vi "运维调试_总氮.vi"() -> ()   [LabVIEW 2016, in "斯坦道总氮.lvlib"]
uses:
  <vilib>/Utility/miscctls.llb/LVPointTypeDef.ctl
  <vilib>/Utility/config.llb/NI_LVConfig.lvlib
  <vilib>/ptbypt/NI_PtbyPt.lvlib
panel:
  in  "定时设置":cluster{"启动":bool, "控制命令":T1}(xcontrol)
  out "单位:":T2(ring)
  out "模块版本号":string
  in  "校准按钮":T3
  out "运行状态":T4 {"数据时间:" format="%<%y/%m/%d %H:%M:%S>T"; "仪器时间:" format="%<%y/%m/%d %H:%M:%S>T"}
  out "一级权限":bool
  out "二级权限":bool
  out "输入密码":u32
  out "布尔":bool
  in  "流程固件":bool
  in  "仪器参数设置":bool
  in  "量程参数读取":T5
  in  "模块启用":bool
  in  "串口设置":bool
  in  "公式一键写入":bool
  in  "流程路径":path=path "C:/Users/STD/Documents/斯坦道流程文件/流程.xml"
  in  "曲线模型":cluster{"X^2":dbl, "X":dbl, "B":dbl, "r^2":dbl}(xcontrol)
  out "字符串":string
  in  "质控参数设置":bool
  in  "自动测试量程配置":T6
  out "温度2":sgl
  out "温度1":sgl
  out "ADC":sgl
  out "固件版本号":string
  in  "数组":string[](array[string])
  in  "量程切换阈值写入":bool
  in  "量程切换阈值读取":bool
  in  "参数下拉列表":enum16{"总磷", "总氮"}(ring)=enum."总氮"
  in  "量程下拉列表":enum16{"低量程", "高量程"}(ring)
  in  "测量模式下拉列表":enum16{"水样测量", "零点核查", "跨度核查", "标样核查", "加标回收"}(ring)
  in  "公式":cluster{"X^2":dbl, "X":dbl, "b":dbl}
  in  "写公式":bool
  in  "读公式":bool
  in  "返回":bool
  in  "设置":bool
  out "集成报警信息":string
  in  "停止":bool
  in  "手动启动":bool
  in  "单步测试":bool
  out "F3":sgl format="%#.6f"
  out "F2":sgl format="%#.6f"
  out "F1":sgl format="%#.6f"
  out "F0":sgl format="%#.6f"
  out "多列列表框":i32(listbox)
  # "参数设置"
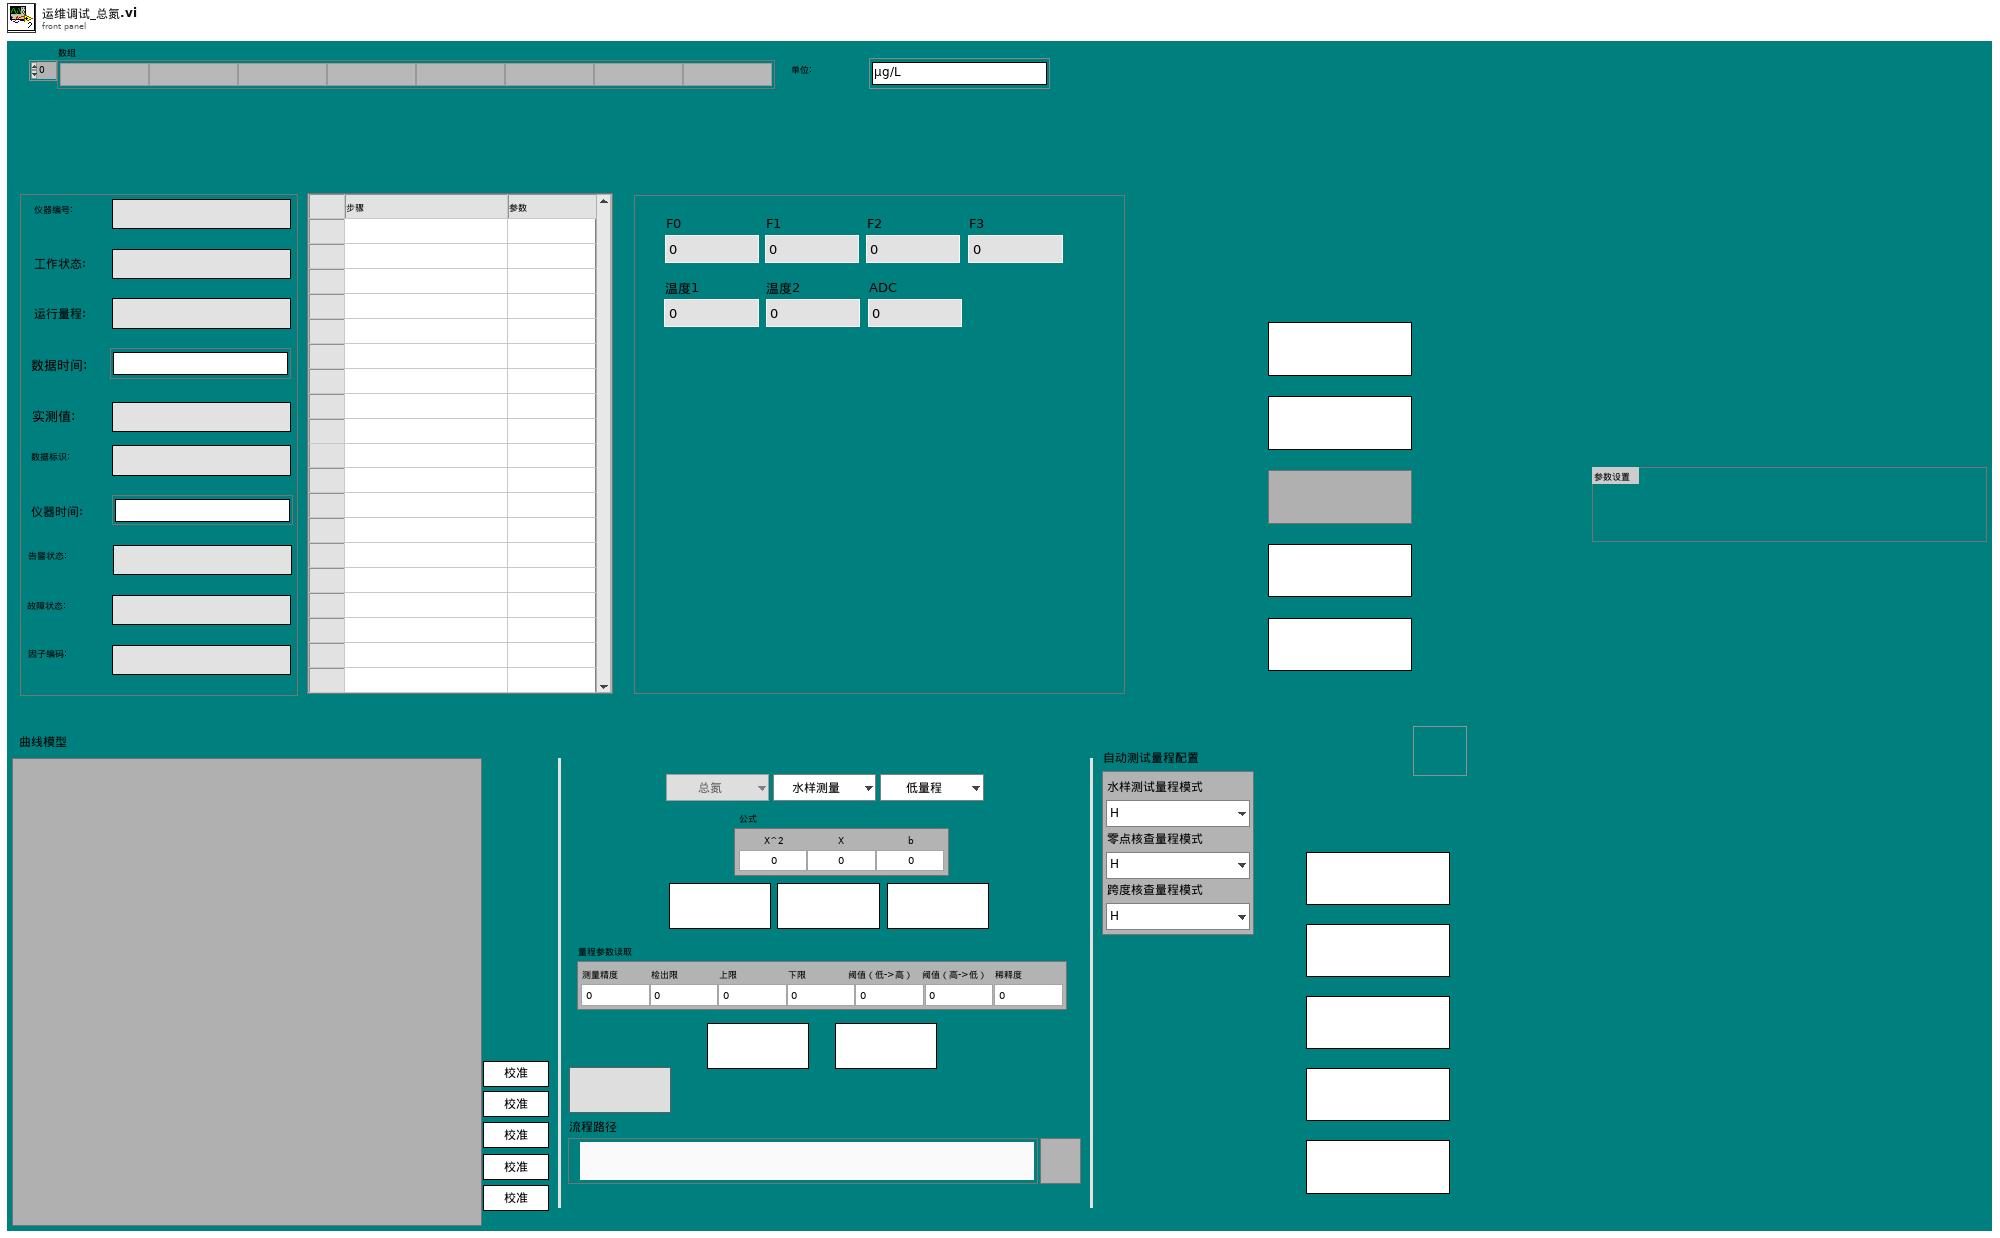
[diagram p1: front panel]
types:
  T1 = typedef "定时设置.xctl/国标控制命令.ctl" = enum16{"启动测量", "标样核查", "零点核查", "跨度核查", "空白测试", "平行样测试", "加标回收", "空白校准", "标样校准", "初始化（清洗）", "停止测试", "仪器重启", "校时", "模式设置", "测量间隔设置"}
  T2 = enum16{"μg/L", "mg/L", "ppm", "mg/m3", "cm", "ppb", "μg/m3", "%", "nmol/mol", "μmol/mol", "MPN/L", "MPN/100ml", "ng/m3", "NTU", "无量纲", "mS/cm", "μS/cm", "℃", "mV", "cells/mL"}
  T3 = cluster{"校准1":bool, "校准2":bool, "校准3":bool, "校准4":bool, "校准5":bool}
  T4 = cluster{"仪器编号:":string, "工作状态:":string, "运行量程: ":string, "数据时间:":timestamp, "实测值:":string, "数据标识: ":string, "仪器时间:":timestamp, "告警状态: ":string, "故障状态:  ":string, "因子编码:":string}
  T5 = cluster{"测量精度":dbl, "检出限":dbl, "上限":dbl, "下限":dbl, "阈值（低->高）":dbl, "阈值（高->低）":dbl, "稀释度":dbl}
  T6 = cluster{"水样测试量程模式":enum16{"H", "L", "AUTO"}, "空白核查量程模式":enum16{"H", "L", "AUTO"}, "跨度核查量程模式":enum16{"H", "L", "AUTO"}}
  T7 = typedef "LVPointTypeDef.ctl" = cluster{"Horizontal":i16, "Vertical":i16}
  T8 = cluster{"系统时间":timestamp, "工作状态":enum16{"空闲", "水样测试", "标样核查", "零点核查", "跨度核查", "空白测试", "平行样测试", "加标回收", "空白校准", "标样校准", "初始化（清洗）"}, "测量模式":enum16{"待机", "连续模式", "周期模式", "定点模式", "受控模式", "手动模式"}, "告警代码":u16, "故障代码":u16, "日志代码":u16, "软件版本":u16, "F0":sgl, "F1":sgl, "F2":sgl, "F3":sgl, "T":sgl, "H":sgl, "id":u16, "flowid":u16, "量程":u16, "总磷控温温度1":sgl, "营养盐控温温度2":sgl, "ADC":sgl}
  T9 = cluster{"因子编码":u32, "单位":u16, "标样参考值":sgl, "水样数据时间":timestamp, "水样实测值":sgl, "水样数据标识":string, "标样数据时间":timestamp, "标样实测值":sgl, "标样数据标识":string, "空白数据时间":timestamp, "空白实测值":sgl, "空白数据标识":string, "零点核查数据时间":timestamp, "零点核查实测值":sgl, "零点核查数据标识":string, "跨度核查数据时间":timestamp, "跨度核查实测值":sgl, "跨度核查数据标识":string, "加标回收数据时间":timestamp, "加标回收实测值":sgl, "加标回收数据标识":string, "平行样数据时间":timestamp, "平行样实测值":sgl, "平行样数据标识":string, "F0":sgl, "F1":sgl, "F2":sgl, "F3":sgl, "F4":sgl, "F5":sgl, "F6":sgl, "F7":sgl, "温度":sgl, "湿度":sgl, "X值":sgl, "fidrange":u16}
  T10 = enum16{"空闲", "水样测试", "标样核查", "零点核查", "跨度核查", "空白测试", "平行样测试", "加标回收", "空白校准", "标样校准", "初始化（清洗）"}
  T11 = enum8{"Enabled", "Disabled", "Disabled and Grayed Out"}
  T12 = cluster{"参数下拉列表":enum16{"总磷", "总氮"}, "测量模式下拉列表":enum16{"水样测量", "零点核查", "跨度核查", "标样核查", "加标回收"}, "量程下拉列表":enum16{"低量程", "高量程"}}
  T13 = cluster{"Major":u16, "Minor":u16, "Fix":u16, "Build":u16}
  T14 = typedef "NI_LVConfig.lvlib/Config Data RefNum.ctl" = refnum<k1>
  T15 = cluster{"启动模式":enum16{"跨度核查", "水样测量", "空白核查", "标样核查", "加标回收"}, "启动参数":u16, "量程":enum16{"低量程", "高量程"}}
  T16 = cluster{"时间标识":timestamp, "设备":string, "日志信息":string, "流程参数":string}
  T17 = typedef "LVRowAndColumnUnsignedTypeDef.ctl" = cluster{"Row":u32, "Column":u32}
  T18 = cluster{"站号":u16, "量程切换":enum32{"H", "L", "AUTO"}, "控制命令":enum16{"启动测量", "标样核查", "零点核查", "跨度核查", "空白测试", "平行样测试", "加标回收", "空白校准", "标样校准", "初始化（清洗）", "停止测试", "仪器重启", "校时", "模式设置", "测量间隔设置"}, "模式设置":enum16{"待机", "连续模式", "周期模式", "定点模式", "受控模式", "手动模式"}, "测量间隔":u16}
  T19 = cluster{"跨度值":dbl, "零点标准液浓度":dbl, "跨度标准液浓度":dbl, "标准液标准浓度":dbl}
  T20 = cluster{"确定":bool, "跨度值":dbl, "零点标准液浓度":dbl, "跨度标准液浓度":dbl, "标准液标准浓度":dbl}
  T21 = cluster{"测量量程":dbl, "测量精度":dbl, "测量间隔":dbl, "消解温度":dbl, "消解时长":dbl, "空白校准时间":timestamp, "曲线截距":dbl, "曲线斜率":dbl, "测量检出限":dbl, "测量信号值":dbl, "线性相关系数":dbl, "二次多项式系数":dbl, "标样校准时间":timestamp, "稀释倍数":dbl, "三项式系数":dbl, "空白标定系数":dbl, "量程系数":dbl, "F0/ORPA":dbl, "F1/ORPB":dbl, "F2/ORPK":dbl, "F3":dbl, "F4":dbl, "F5":dbl, "F6":dbl, "F7":dbl, "X0/滴定数":dbl, "量程":dbl}
  T22 = cluster{"确定":bool, "测量量程":dbl, "测量精度":dbl, "测量间隔":dbl, "消解温度":dbl, "消解时长":dbl, "空白校准时间":timestamp, "曲线截距":dbl, "曲线斜率":dbl, "测量检出限":dbl, "测量信号值":dbl, "线性相关系数":dbl, "二次多项式系数":dbl, "标样校准时间":timestamp, "稀释倍数":dbl, "三项式系数":dbl, "空白标定系数":dbl, "量程系数":dbl, "F0/ORPA":dbl, "F1/ORPB":dbl, "F2/ORPK":dbl, "F3":dbl, "F4":dbl, "F5":dbl, "F6":dbl, "F7":dbl, "X0/滴定数":dbl, "量程":dbl}
  T23 = cluster{"标液浓度1":dbl, "标液浓度2":dbl, "标液浓度3":dbl, "标液浓度4":dbl, "标液浓度5":dbl}
  T24 = cluster{"测量精度":u16, "检出限":dbl, "上限":dbl, "下限":dbl, "阈值（低->高）":dbl, "阈值（高->低）":dbl, "稀释度":dbl}
  T25 = enum32{"Bad", "Idle", "Run top level", "Running"}
  T26 = typedef "定时设置.xctl/周期模式设置.ctl" = enum16{"不启用", "定点模式", "间隔模式"}
  T27 = typedef "定时设置.xctl/定点周期设置.ctl" = cluster{"启动命令":T28, "启动命令 2":T28, "启动命令 3":T28, "启动命令 4":T28, "启动命令 5":T28, "启动命令 6":T28, "启动命令 7":T28, "启动命令 8":T28, "启动命令 9":T28, "启动命令 10":T28, "启动命令 11":T28, "启动命令 12":T28, "启动命令 13":T28, "启动命令 14":T28, "启动命令 15":T28, "启动命令 16":T28, "启动命令 17":T28, "启动命令 18":T28, "启动命令 19":T28, "启动命令 20":T28, "启动命令 21":T28, "启动命令 22":T28, "启动命令 23":T28, "启动命令 24":T28}
  T28 = typedef "定时设置.xctl/启动命令选择.ctl" = u16
  T29 = typedef "定时设置.xctl/间隔启动设置.ctl" = cluster{"启动命令":T28, "启动间隔":dbl, "启动次数":i32}
  T30 = cluster{"时间标识":timestamp, "设备":string, "日志信息":string, "备注":string}
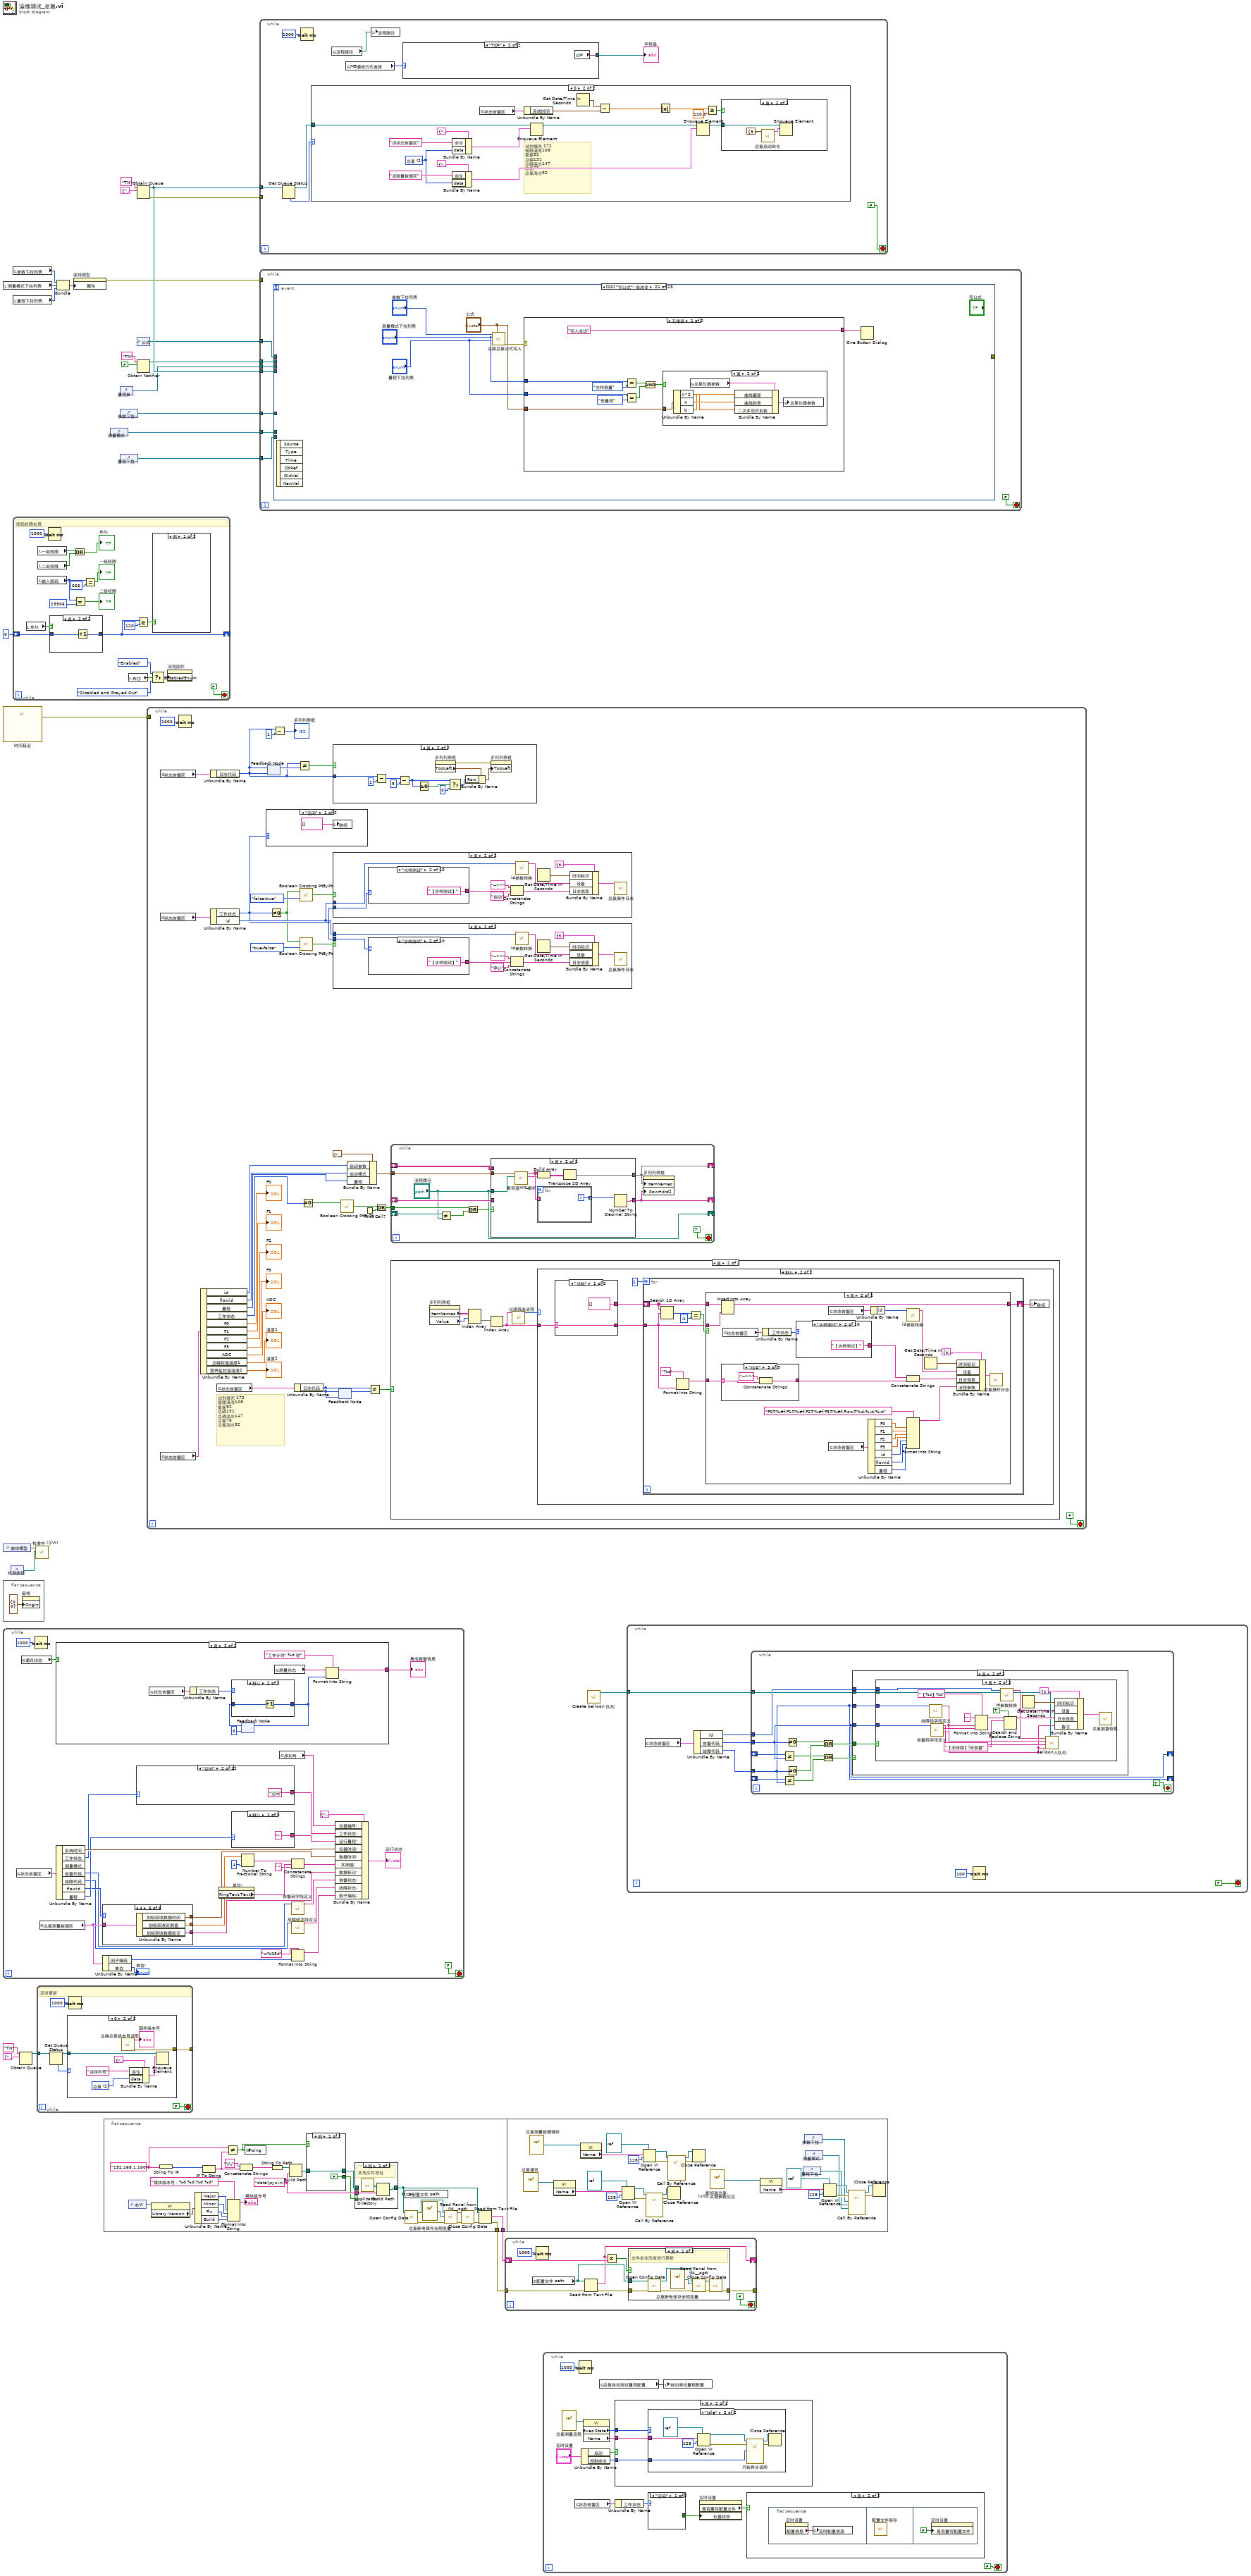
[diagram p0: block diagram]
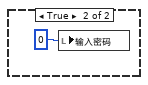
[diagram p5: hidden frame]
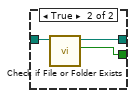
[diagram p7: hidden frame]
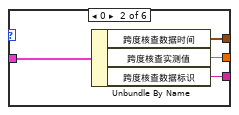
[diagram p11: hidden frame]
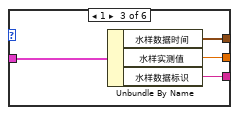
[diagram p12: hidden frame]
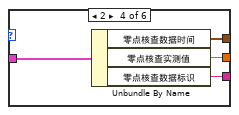
[diagram p13: hidden frame]
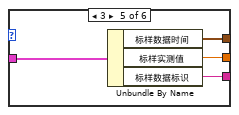
[diagram p14: hidden frame]
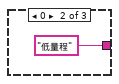
[diagram p15: hidden frame]
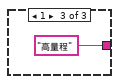
[diagram p16: hidden frame]
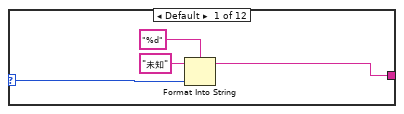
[diagram p17: hidden frame]
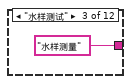
[diagram p18: hidden frame]
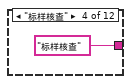
[diagram p19: hidden frame]
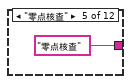
[diagram p20: hidden frame]
diagram:
  n1 = local read "测量模式下拉列表"() -> (w9:enum16{"水样测量", "零点核查", "跨度核查", "标样核查", "加标回收"})
  n2 = call "时间延迟"() -> ("error out"=w19:errorcluster)  [unwired: 11 in]
  n3 = control-ref of="曲线模型"() -> (w4:refnum<vi>)
  n4 = flat-sequence {
    frame #0 {
      n5 = property on="窗格" class="Pane"("Origin"=T7 {"Horizontal"=0, "Vertical"=0} ("原点")) -> ()  [unwired: 2 in, 2 out]
    }
  }
  n6 = while {
    stop <- FALSE stop-if-true
    n7 = global read "VAR总氮全局变量.vi" "状态告警区"() -> (w49:T8)
    n8 = global read "VAR总氮全局变量.vi" "通讯状态"() -> (w57:bool)
    n9 = Wait (ms)(milliseconds to wait=u32 1000 ("等待时间（毫秒）")) -> ()  [unwired: 1 out]
    n10 = global read "VAR总氮全局变量.vi" "总氮测量数据区"() -> (w46:T9)
    n11 = case shown="真" w57 {
      tunnel: ["通讯异常" ("集成报警信息") w100] -> w56
      frame False {
      }
      frame True {
        n12 = global read "VAR总氮全局变量.vi" "状态告警区"() -> (w106:T8)
        n13 = Unbundle By Name(w106) -> ("工作状态"=w105:T10)
        n14 = feedback #1(0) -> (w103:i32)
        n15 = case shown="默认" w105 {
          tunnel: w103 -> [_ w108]
          tunnel: [_ w107] -> w101
          frame "空闲" {
          }
          frame Default {
            n16 = Increment(x=w108) -> (x+1=w107:i32)
          }
        }
        n17 = feedback-in #1(w101) -> ()
        n18 = global read "VAR总氮全局变量.vi" "测量状态"() -> (w99:string)
        n19 = Format Into String(format string="工作计时: %d 秒" ("格式字符串"), initial string=w99, w101) -> (resulting string=w100:string)  [unwired: 1 in, 1 out]
      }
    }
    "集成报警信息" <- w56
    n20 = Unbundle By Name(w49) -> ("系统时间"=w55:timestamp, "工作状态"=w47:T10, "告警代码"=w32:u16, "故障代码"=w30:u16, "flowid"=w45:u16, "量程"=w53:u16)  [unwired: 1 out]
    n21 = case shown="4" w45 {
      tunnel: [_ w63 w67 w71 w75 w79] -> w41
      tunnel: [_ w61 w66 w70 w74 w78] -> w37
      tunnel: [_ w60 w65 w69 w73 w77] -> w34
      tunnel: w46 -> [_ w62 w64 w68 w72 w76]
      frame Default {
      }
      frame 0 {
        n22 = Unbundle By Name(w62) -> ("跨度核查数据时间"=w63:timestamp, "跨度核查实测值"=w61:sgl, "跨度核查数据标识"=w60:string)
      }
      frame 1 {
        n23 = Unbundle By Name(w64) -> ("水样数据时间"=w67:timestamp, "水样实测值"=w66:sgl, "水样数据标识"=w65:string)
      }
      frame 2 {
        n24 = Unbundle By Name(w68) -> ("零点核查数据时间"=w71:timestamp, "零点核查实测值"=w70:sgl, "零点核查数据标识"=w69:string)
      }
      frame 3 {
        n25 = Unbundle By Name(w72) -> ("标样数据时间"=w75:timestamp, "标样实测值"=w74:sgl, "标样数据标识"=w73:string)
      }
      frame 4 {
        n26 = Unbundle By Name(w76) -> ("加标回收数据时间"=w79:timestamp, "加标回收实测值"=w78:sgl, "加标回收数据标识"=w77:string)
      }
    }
    n27 = Unbundle By Name(w46) -> ("因子编码"=w50:u32, "单位"=→"单位:":u16)
    n28 = case shown="\"空闲\"" w47 {
      selector: w47 -> [w83 _ _ _ _ _ _ _ _ _ _ _]
      tunnel: [w84 "空闲" ("工作状态") "水样测量" ("工作状态") "标样核查" ("工作状态") "零点核查" ("工作状态") "跨度核查" ("工作状态") "空白测试" ("工作状态") "平行样测试" ("工作状态") "加标回收" ("工作状态") "空白校准" ("工作状态") "标样校准" ("工作状态") "初始化" ("工作状态")] -> w54
      frame Default {
        n29 = Format Into String(format string="%d" ("格式字符串"), initial string="未知" ("工作状态"), w83) -> (resulting string=w84:string)  [unwired: 1 in, 1 out]
      }
      frame "空闲" {
      }
      frame "水样测试" {
      }
      frame "标样核查" {
      }
      frame "零点核查" {
      }
      frame "跨度核查" {
      }
      frame "空白测试" {
      }
      frame "平行样测试" {
      }
      frame "加标回收" {
      }
      frame "空白校准" {
      }
      frame "标样校准" {
      }
      frame "初始化（清洗）" {
      }
    }
    n30 = property on="单位:" class="Enum (严格)"() -> ("RingText.Text"=w38:string)  [unwired: 2 in, 2 out]
    n31 = case shown="默认" w53 {
      tunnel: ["" ("字符串") "低量程" ("字符串") "高量程" ("字符串")] -> w52
      frame Default {
      }
      frame 0 {
      }
      frame 1 {
      }
    }
    n32 = Number To Fractional String(number=w37, precision (6)=i16 4 ("精度(6)")) -> (F-format string=w36:string)  [unwired: 2 in]
    n33 = global read "VAR总氮全局变量.vi" "序列号"() -> (w48:string)
    n34 = Concatenate Strings(w36, " " ("字符串"), w38) -> (w35:string)
    n35 = call "告警码字段定义.vi"("告警代码"=w32) -> ("字符串"=w31:string)  [unwired: 8 in, 2 out]
    n36 = call "故障码字段定义.vi"("故障代码"=w30) -> ("字符串"=w29:string)  [unwired: 10 in]
    n37 = Format Into String(format string="w%05d" ("格式字符串"), w50) -> (resulting string=w33:string)  [unwired: 2 in, 1 out]
    n38 = Bundle By Name(cluster=T4 {"仪器编号:"="", "工作状态:"="", "运行量程: "="", "数据时间:"=timestamp(0 s since 1904-01-01), "实测值:"="", "数据标识: "="", "仪器时间:"=timestamp(0 s since 1904-01-01), "告警状态: "="", "故障状态:  "="", "因子编码:"=""} ("运行状态"), "仪器编号:"=w48, "工作状态:"=w54, "运行量程:"=w52, "仪器时间:"=w55, "数据时间:"=w41, "实测值:"=w35, "数据标识:"=w34, "告警状态:"=w31, "故障状态:"=w29, "因子编码:"=w33) -> (→"运行状态":T4)
  }
  n39 = control-ref of="校准按钮"() -> (w3:refnum<vi>)
  n40 = local read "参数下拉列表"() -> (w10:enum16{"总磷", "总氮"})
  n41 = local read "量程下拉列表"() -> (w8:enum16{"低量程", "高量程"})
  n42 = while {
    shift-right: [w115] -> _
    shift-left: u32 0 ("等待时间（毫秒）") -> [w116]
    stop <- FALSE stop-if-true
    # "密码权限处理"
    n43 = local read "布尔"() -> (w117:bool)
    n44 = local read "一级权限"() -> (w119:bool)
    n45 = local read "二级权限"() -> (w120:bool)
    n46 = local read "输入密码"() -> (w123:u32)
    n47 = Wait (ms)(milliseconds to wait=u32 1000 ("等待时间（毫秒）")) -> ()  [unwired: 1 out]
    n48 = case shown="真" w117 {
      tunnel: w116 -> [_ w130]
      tunnel: [_ w129] -> w115
      frame False {
      }
      frame True {
        n49 = Increment(x=w130) -> (x+1=w129:u32)
      }
    }
    n50 = Or(x=w119, y=w120) -> (x .or. y?=→"布尔":bool)
    n51 = Equal?(x=w123, y=u32 23506) -> (x = y?=→"二级权限":bool)
    n52 = Equal?(x=w123, y=u32 666) -> (x = y?=→"一级权限":bool)
    n53 = local read "布尔"() -> (w112:bool)
    n54 = Greater Or Equal?(x=w115, y=u32 120) -> (x >= y?=w113:bool)
    n55 = Select(t=T11."Enabled" ("禁用"), s=w112, f=T11."Disabled and Grayed Out") -> (s? t:f=w110:T11)
    n56 = case shown="假" w113 {
      frame False {
      }
      frame True {
        n57 = local write "输入密码"(u32 0 ("输入密码")) -> ()
      }
    }
    n58 = property on="流程固件" class="Bool"("DisabledEnum"=w110) -> ()  [unwired: 2 in, 2 out]
  }
  n59 = Obtain Queue(name (unnamed)="TN" ("名称（未命名）"), element data type=cluster{"命令":string, "data":variant} {"命令"="", "data"=variant}) -> (queue out=w16:refnum<queue>)  [unwired: 3 in, 2 out]
  n60 = call "校准中 (子VI).vi"("曲线模型"=w4, "校准按钮"=w3) -> ()  [unwired: 9 in]
  n61 = while {
    tunnel: w16 -> [w135]
    tunnel: [w133] -> _
    stop <- FALSE stop-if-true
    # "定时更新"
    n62 = Get Queue Status(queue=w135) -> (queue out=w132:refnum<queue>, # elements in queue=w131:i32)  [unwired: 2 in, 6 out]
    n63 = case shown="0" w131 {
      tunnel: [_ w138] -> w133
      tunnel: w132 -> [_ w137]
      frame Default {
      }
      frame 0 {
        w141 = u16 2 items=["总磷"=1, "总氮"=2, "氨氮"=3] ("站号")
        n64 = call "总磷总氮版本号读取.vi"() -> ("error out"=w138:errorcluster, "固件版本号"=→"固件版本号":string)  [unwired: 10 in]
        n65 = Bundle By Name(cluster=cluster{"命令":string, "data":variant} {"命令"="", "data"=variant} ("元素"), "命令"="读序列号", "data"=w141) -> (w140:cluster{"命令":string, "data":variant})
        n66 = Enqueue Element(queue=w137, element=w140) -> ()  [unwired: 2 in, 3 out]
      }
    }
    n67 = Wait (ms)(milliseconds to wait=u32 1000 ("等待时间（毫秒）")) -> ()  [unwired: 1 out]
  }
  n68 = Bundle("参数下拉列表"=w10, "测量模式下拉列表"=w9, "量程下拉列表"=w8) -> (w7:T12)  [unwired: 1 in]
  n69 = property on="曲线模型" class="曲线模型 (严格)"("属性"=w7) -> (error out=w15:errorcluster)  [unwired: 2 in, 1 out]
  n70 = flat-sequence {
    tunnel: [w153] -> w1
    tunnel: [w152] -> w5
    frame #0 {
      w166 = "data\\sys.ini" ("名称或相对路径")
      w158 = "192.168.1.100" ("名称")
      n71 = control-ref of="本VI"() -> (w151:refnum<vi>)
      n72 = property class="VI"(reference=w151) -> ("Library.Version"=w150:T13)  [unwired: 1 in, 2 out]
      n73 = String To IP(1:w158) -> (0:w165:u32)
      n74 = Unbundle By Name(w150) -> ("Major"=w148:u16, "Minor"=w147:u16, "Fix"=w146:u16, "Build"=w145:u16)
      n75 = IP To String(2:w165) -> (0:w162:string)  [unwired: 1 in]
      n76 = Not Equal?(x=w158, y=w162) -> (x != y?=w156:bool)
      n77 = Format Into String(format string="模块版本号：%d.%d.%d.%d" ("格式字符串"), w148, w147, w146, w145) -> (resulting string=→"模块版本号":string)  [unwired: 2 in, 1 out]
      n78 = Concatenate Strings("\\\\" ("字符串"), w162) -> (w163:string)
      n79 = global write "VAR总氮全局变量.vi" "ping"(w156) -> ()
      n80 = String To Path(string=w163) -> (path=w157:path)
      n81 = Build Path(base path=w157, name or relative path=w166) -> (appended path=w161:path)
      n82 = case shown="假" w156 {
        tunnel: w161 -> [w172 w176]
        tunnel: [w172 w175] -> w160
        tunnel: [FALSE w174] -> w159
        frame False {
        }
        frame True {
          n83 = call <vilib>:"Check if File or Folder Exists.vi"("path"=w176) -> ("file or folder exists?"=w174:bool, "dup path"=w175:path)  [unwired: 8 in, 1 out]
        }
      }
      n84 = case shown="假" w159 {
        tunnel: w160 -> [_ w180]
        tunnel: [w178 w180] -> w155
        tunnel: w166 -> [w177 _]
        frame False {
          # "本地文件地址"
          n85 = call <vilib>:"Application Directory.vi"() -> ("Application Directory"=w179:path)
          n86 = Build Path(base path=w179, name or relative path=w177) -> (appended path=w178:path)
        }
        frame True {
          # "网络共享地址"
        }
      }
      n87 = global write "VAR总氮全局变量.vi" "配置文件 path"(w155) -> ()
      n88 = call <vilib>:"Open Config Data.vi"("configuration file path"=w155) -> ("error out"=w168:errorcluster, "refnum"=w171:T14)  [unwired: 8 in, 1 out]
      n89 = vi-ref "总氮断电保存全局变量.vi"() -> (w170:refnum<vi>)
      n90 = call <userlib>:"Read Panel from INI__ogtk.vi"("error in (no error)"=w168, "VI ref"=w170, "refnum"=w171) -> ("error out"=w167:errorcluster, "refnum out"=w169:T14)  [unwired: 7 in]
      n91 = call <vilib>:"Close Config Data.vi"("error in (no error)"=w167, "refnum"=w169) -> ("error out"=w154:errorcluster)  [unwired: 8 in, 1 out]
      n92 = Read from Text File(file (use dialog)=w155, error in=w154) -> (text=w152:string, error out=w153:errorcluster)  [unwired: 2 in, 2 out]
    }
    frame #1 {
      n93 = vi-ref "总氮通讯.vi"() -> (w207:refnum<vi>)
      n94 = vi-ref "总氮测量数据储存.vi"() -> (w199:refnum<vi>)
      n95 = property class="VI"(reference=w207) -> ("Name"=w206:string)  [unwired: 1 in, 2 out]
      n96 = property class="VI"(reference=w199) -> ("Name"=w192:string)  [unwired: 1 in, 2 out]
      n97 = Open VI Reference(type specifier VI Refnum (for type only)=refnum<vi> refnum, vi path=w206, options=128 ("选项")) -> (vi reference=w204:refnum<vi>, error out=w202:errorcluster)  [unwired: 3 in]
      n98 = Open VI Reference(type specifier VI Refnum (for type only)=refnum<vi> refnum, vi path=w192, options=128 ("选项")) -> (vi reference=w194:refnum<vi>, error out=w196:errorcluster)  [unwired: 3 in]
      n99 = call-by-ref "?"(reference=w204, error in=w202) -> (reference out=w200:refnum<vi>, error out=w201:errorcluster)  [unwired: 12 in]
      n100 = call-by-ref "?"(reference=w194, error in=w196) -> (reference out=w198:refnum<vi>, error out=w197:errorcluster)  [unwired: 12 in]
      n101 = Close Reference(reference=w200, error in (no error)=w201) -> ()  [unwired: 1 out]
      n102 = Close Reference(reference=w198, error in (no error)=w197) -> ()  [unwired: 1 out]
      n103 = vi-ref "斯坦道总氮.lvlib:关键参数交互.vi"() -> (w184:refnum<vi>)
      n104 = property class="VI"(reference=w184) -> ("Name"=w191:string)  [unwired: 1 in, 2 out]
      n105 = control-ref of="量程下拉列表"() -> (w181:refnum<vi>)
      n106 = control-ref of="参数下拉列表"() -> (w183:refnum<vi>)
      n107 = control-ref of="测量模式下拉列表"() -> (w182:refnum<vi>)
      n108 = Open VI Reference(type specifier VI Refnum (for type only)=refnum<vi> refnum, vi path=w191, options=128 ("选项")) -> (vi reference=w189:refnum<vi>, error out=w187:errorcluster)  [unwired: 3 in]
      n109 = call-by-ref "?"(reference=w189, error in=w187, "量程下拉列表"=w181, "测量模式下拉列表"=w182, "测量参数"=w183) -> (reference out=w185:refnum<vi>, error out=w186:errorcluster)  [unwired: 9 in]
      n110 = Close Reference(reference=w185, error in (no error)=w186) -> ()  [unwired: 1 out]
    }
  }
  n111 = control-ref of="测量模式下拉列表"() -> (w21:refnum<vi>)
  n112 = control-ref of="量程参数读取"() -> (w11:refnum<vi>)
  n113 = control-ref of="参数下拉列表"() -> (w22:refnum<vi>)
  n114 = control-ref of="量程下拉列表"() -> (w23:refnum<vi>)
  n115 = Obtain Queue(name (unnamed)="TN" ("名称（未命名）"), element data type=cluster{"命令":string, "data":variant} {"命令"="", "data"=variant}) -> (queue out=w24:refnum<queue>, error out=w25:errorcluster)  [unwired: 3 in, 1 out]
  n116 = control-ref of="公式"() -> (w20:refnum<vi>)
  n117 = Obtain Notifier(name (unnamed)="TN" ("名称（未命名）"), notification data type=FALSE) -> (notifier out=w12:refnum<notifier>)  [unwired: 2 in, 2 out]
  n118 = while {
    tunnel: w19 -> [_]
    stop <- FALSE stop-if-true
    # "试剂填充 172 \n管路清洗108\n氨氮92\n总磷131\n总磷海水147\n总氮76\n总氮海水92"
    n119 = global read "VAR总氮全局变量.vi" "状态告警区"() -> (w230:T8)
    n120 = global read "VAR总氮全局变量.vi" "状态告警区"() -> (w228:T8)
    n121 = global read "VAR总氮全局变量.vi" "状态告警区"() -> (w238:T8)
    n122 = Wait (ms)(milliseconds to wait=u32 1000 ("等待时间（毫秒）")) -> ()  [unwired: 1 out]
    n123 = Unbundle By Name(w238) -> ("id"=w235:u16, "flowid"=w237:u16, "量程"=w236:u16, "工作状态"=w216:T10, "F0"=→"F0":sgl, "F1"=→"F1":sgl, "F2"=→"F2":sgl, "F3"=→"F3":sgl, "ADC"=→"ADC":sgl, "总磷控温温度1"=→"温度1":sgl, "营养盐控温温度2"=→"温度2":sgl)
    n124 = Unbundle By Name(w230) -> ("日志代码"=w222:u16)
    n125 = Unbundle By Name(w228) -> ("工作状态"=w208:T10, "id"=w212:u16)
    n126 = global read "VAR总氮全局变量.vi" "状态告警区"() -> (w226:T8)
    n127 = case shown="\"空闲\"" w208 {
      frame "空闲" {
        n128 = local write "数组"(string[] [] ("数组")) -> ()
      }
      frame "水样测试", Default {
      }
    }
    n129 = feedback-in #2(w222) -> ()
    n130 = feedback #2(w222) -> (w243:u16)
    n131 = Not Equal To 0?(x=w208) -> (x != 0?=w210:bool)
    n132 = Subtract(x=w222, y=1) -> (x-y=→"多列列表框":i32)
    n133 = Unbundle By Name(w226) -> ("日志代码"=w225:u16)
    n134 = Not Equal?(x=w222, y=w243) -> (x != y?=w242:bool)
    n135 = call <vilib>:"Boolean Crossing PtByPt.vi"("direction"=enum16{"either", "false-true", "true-false"}."false-true", "input"=w210) -> ("crossing"=w214:bool)  [unwired: 1 in]
    n136 = call <vilib>:"Boolean Crossing PtByPt.vi"("direction"=enum16{"either", "false-true", "true-false"}."true-false", "input"=w210) -> ("crossing"=w209:bool)  [unwired: 1 in]
    n137 = Not Equal To 0?(x=w216) -> (x != 0?=w240:bool)
    n138 = case shown="真" w242 {
      tunnel: w222 -> [_ w373]
      frame False {
      }
      frame True {
        n139 = Subtract(x=w373, y=1) -> (x-y=w371:i32)
        n140 = Subtract(x=w371, y=5) -> (x-y=w375:i32)
        n141 = Greater Or Equal To 0?(x=w375) -> (x >= 0?=w374:bool)
        n142 = property on="多列列表框" class="MCListbox (严格)"() -> (error out=w379:errorcluster, "TopLeft"=w380:T17)  [unwired: 2 in, 1 out]
        n143 = Select(t=w375, s=w374, f=0) -> (s? t:f=w376:i32)
        n144 = Bundle By Name(cluster=w380, "Row"=w376) -> (w381:T17)
        n145 = property on="多列列表框" class="MCListbox (严格)"(error in=w379, "TopLeft"=w381) -> ()  [unwired: 1 in, 2 out]
      }
    }
    n146 = case shown="真" w214 {
      tunnel: w212 -> [_ w265]
      tunnel: w208 -> [_ w269]
      frame False {
      }
      frame True {
        n147 = case shown="\"水样测试\"" w269 {
          tunnel: [_ "【水样测试】" ("字符串") "【标样核查】" ("字符串") "【零点核查】" ("字符串") "【跨度核查】" ("字符串") "【空白测试】" ("字符串") "【平行样测试】" ("字符串") "【加标回收】" ("字符串") "【空白校准】" ("字符串") "【标样校准】" ("字符串")] -> w273
          frame "空闲", Default {
          }
          frame "水样测试" {
          }
          frame "标样核查" {
          }
          frame "零点核查" {
          }
          frame "跨度核查" {
          }
          frame "空白测试" {
          }
          frame "平行样测试" {
          }
          frame "加标回收" {
          }
          frame "空白校准" {
          }
          frame "标样校准" {
          }
        }
        n148 = Concatenate Strings("-->>" ("字符串"), w273, "启动" ("字符串")) -> (w274:string)
        n149 = call "id参数转换.vi"("id"=w265) -> ("table输出"=w266:string)  [unwired: 10 in]
        n150 = Get Date/Time In Seconds() -> (seconds since 1Jan1904=w271:timestamp)
        n151 = Bundle By Name(cluster=T16 {"时间标识"=timestamp(0 s since 1904-01-01), "设备"="", "日志信息"="", "流程参数"=""} ("data in"), "时间标识"=w271, "设备"=w266, "日志信息"=w274) -> (w270:T16)
        n152 = call "总氮操作日志.vi"("data in"=w270) -> ()  [unwired: 11 in]
      }
    }
    n153 = case shown="真" w209 {
      tunnel: w212 -> [_ w246]
      tunnel: w208 -> [_ w250]
      frame False {
      }
      frame True {
        n154 = case shown="\"水样测试\"" w250 {
          tunnel: [_ "【水样测试】" ("字符串") "【标样核查】" ("字符串") "【零点核查】" ("字符串") "【跨度核查】" ("字符串") "【空白测试】" ("字符串") "【平行样测试】" ("字符串") "【加标回收】" ("字符串") "【空白校准】" ("字符串") "【标样校准】" ("字符串")] -> w254
          frame "空闲", Default {
          }
          frame "水样测试" {
          }
          frame "标样核查" {
          }
          frame "零点核查" {
          }
          frame "跨度核查" {
          }
          frame "空白测试" {
          }
          frame "平行样测试" {
          }
          frame "加标回收" {
          }
          frame "空白校准" {
          }
          frame "标样校准" {
          }
        }
        n155 = Concatenate Strings("-->>" ("字符串"), w254, "停止" ("字符串")) -> (w255:string)
        n156 = call "id参数转换.vi"("id"=w246) -> ("table输出"=w247:string)  [unwired: 10 in]
        n157 = Get Date/Time In Seconds() -> (seconds since 1Jan1904=w252:timestamp)
        n158 = Bundle By Name(cluster=T16 {"时间标识"=timestamp(0 s since 1904-01-01), "设备"="", "日志信息"="", "流程参数"=""} ("data in"), "时间标识"=w252, "设备"=w247, "日志信息"=w255) -> (w251:T16)
        n159 = call "总氮操作日志.vi"("data in"=w251) -> ()  [unwired: 11 in]
      }
    }
    n160 = feedback #3(w225) -> (w227:u16)
    n161 = feedback-in #3(w225) -> ()
    n162 = call <vilib>:"Boolean Crossing PtByPt.vi"("input"=w240) -> ("crossing"=w215:bool)  [unwired: 2 in]
    n163 = Bundle By Name(cluster=T15 {"启动模式"=enum."跨度核查", "启动参数"=1, "量程"=enum."低量程"} ("参数簇"), "启动参数"=w235, "启动模式"=w237, "量程"=w236) -> (w229:T15)
    n164 = First Call?() -> (First Call?: T/F=w241:bool)
    n165 = Not Equal?(x=w225, y=w227) -> (x != y?=w224:bool)
    n166 = Or(x=w215, y=w241) -> (x .or. y?=w239:bool)
    n167 = while {
      tunnel: w239 -> [w359]
      tunnel: w229 -> [w358]
      shift-right: [w353] -> _
      shift-left: _ -> [w355]
      shift-right: [w354] -> _
      shift-left: _ -> [w356]
      shift-right: ["流程路径"] -> _
      shift-left: _ -> [w352]
      stop <- TRUE stop-if-true
      n168 = Not Equal?(x=w352, y="流程路径") -> (x != y?=w349:bool)
      n169 = Or(x=w359, y=w349) -> (x .or. y?=w350:bool)
      n170 = case shown="真" w350 {
        tunnel: [w361 w369] -> w354
        tunnel: [w360 w368] -> w353
        tunnel: w358 -> [_ w363]
        tunnel: w356 -> [w361 _]
        tunnel: w355 -> [w360 _]
        tunnel: "流程路径" -> [_ w362]
        frame False {
        }
        frame True {
          n171 = call "斯坦道XML解析.vi"("添加的路径"=w362, "参数簇"=w363) -> ("步骤时间"=w364:string[], "步骤名"=w366:string[])  [unwired: 8 in]
          n172 = Build Array(w366, w364) -> (w365:string[][])
          n173 = for {
            tunnel: w366 -> [_] mode=indexing
            tunnel: [w370] -> w367 mode=indexing
            i -> [w370]
          }
          n174 = Transpose 2D Array(2D array=w365) -> (transposed array=w368:string[][])
          n175 = Number To Decimal String(number=w367) -> (decimal integer string=w369:string[])  [unwired: 1 in]
        }
      }
      n176 = property on="多列列表框" class="MCListbox (严格)"("ItemNames"=w353, "RowHdrs[]"=w354) -> ()  [unwired: 2 in, 2 out]
    }
    n177 = case shown="真" w224 {
      frame False {
      }
      frame True {
        n178 = property on="多列列表框" class="MCListbox (严格)"() -> ("ItemNames"=w288:string[][], "Value"=w289:i32)  [unwired: 2 in, 2 out]
        n179 = Index Array(array=w288, index (row)=w289) -> (element=w287:string[])  [unwired: 1 in]
        n180 = Index Array(array=w287) -> (element=w286:string)  [unwired: 1 in]
        n181 = call "过滤筛选流程.vi"("字符串"=w286) -> ("匹配后偏移量"=w285:i32)  [unwired: 10 in]
        n182 = case shown="默认" w285 {
          tunnel: w286 -> [_ w290]
          frame -1 {
          }
          frame Default {
            n183 = case shown="\"读数\"" w290 {
              selector: w290 -> [w296 w298]
              tunnel: [w296 w298] -> w292
              tunnel: [string[] [] ("数组") "数组"] -> w291
              frame "读数" {
              }
              frame Default {
              }
            }
            n184 = for {
              N: 1 -> [_]
              tunnel: w292 -> [w300]
              shift-right: [w299] -> w293
              shift-left: w291 -> [w301]
              n185 = Search 1D Array(1D array=w301, element=w300) -> (index of element=w304:i32)  [unwired: 1 in]
              n186 = Format Into String(format string="%s" ("格式字符串"), w300) -> (resulting string=w305:string)  [unwired: 2 in, 1 out]
              n187 = Equal?(x=w304, y=-1) -> (x = y?=w302:bool)
              n188 = case shown="真" w302 {
                tunnel: w305 -> [_ w315]
                tunnel: w301 -> [w307 w319]
                tunnel: w300 -> [_ w318]
                tunnel: [w307 w317] -> w299
                frame False {
                }
                frame True {
                  n189 = Insert Into Array(array=w319, new element=w318) -> (w317:string[])  [unwired: 1 in]
                  n190 = case shown="\"结束\"" w315 {
                    selector: w315 -> [w342 w345 w348]
                    tunnel: [w342 w344 w347] -> w311
                    frame Default {
                    }
                    frame "初始化" {
                      n191 = Concatenate Strings("-->>" ("字符串"), w345) -> (w344:string)
                    }
                    frame "结束" {
                      n192 = Concatenate Strings("-->>" ("字符串"), w348) -> (w347:string)
                    }
                  }
                  n193 = global read "VAR总氮全局变量.vi" "状态告警区"() -> (w314:T8)
                  n194 = Unbundle By Name(w314) -> ("工作状态"=w313:T10)
                  n195 = case shown="\"水样测试\"" w313 {
                    tunnel: [_ "【水样测试】" ("字符串") "【标样核查】" ("字符串") "【零点核查】" ("字符串") "【跨度核查】" ("字符串") "【空白测试】" ("字符串") "【平行样测试】" ("字符串") "【加标回收】" ("字符串") "【空白校准】" ("字符串") "【标样校准】" ("字符串")] -> w312
                    frame "空闲", Default {
                    }
                    frame "水样测试" {
                    }
                    frame "标样核查" {
                    }
                    frame "零点核查" {
                    }
                    frame "跨度核查" {
                    }
                    frame "空白测试" {
                    }
                    frame "平行样测试" {
                    }
                    frame "加标回收" {
                    }
                    frame "空白校准" {
                    }
                    frame "标样校准" {
                    }
                  }
                  n196 = global read "VAR总氮全局变量.vi" "状态告警区"() -> (w332:T8)
                  n197 = global read "VAR总氮全局变量.vi" "状态告警区"() -> (w329:T8)
                  n198 = Unbundle By Name(w329) -> ("F0"=w326:sgl, "F1"=w325:sgl, "F2"=w324:sgl, "F3"=w323:sgl, "id"=w322:u16, "flowid"=w321:u16, "量程"=w320:u16)
                  n199 = Unbundle By Name(w332) -> ("id"=w309:u16)
                  n200 = call "id参数转换.vi"("id"=w309) -> ("table输出"=w308:string)  [unwired: 10 in]
                  n201 = Concatenate Strings(w312, w311) -> (w310:string)
                  n202 = Format Into String(format string="F0=%#f,F1=%#f,F2=%#f,F3=%#f,Flow=%d-%-d-%-d" ("格式字符串"), w326, w325, w324, w323, w322, w321, w320) -> (resulting string=w327:string)  [unwired: 2 in, 1 out]
                  n203 = Get Date/Time In Seconds() -> (seconds since 1Jan1904=w330:timestamp)
                  n204 = Bundle By Name(cluster=T16 {"时间标识"=timestamp(0 s since 1904-01-01), "设备"="", "日志信息"="", "流程参数"=""} ("data in"), "时间标识"=w330, "设备"=w308, "日志信息"=w310, "流程参数"=w327) -> (w331:T16)
                  n205 = call "总氮操作日志.vi"("data in"=w331) -> ()  [unwired: 11 in]
                }
              }
            }
            n206 = local write "数组"(w293) -> ()
          }
        }
      }
    }
  }
  n207 = while {
    tunnel: w24 -> [w387]
    tunnel: w25 -> [_]
    stop <- FALSE stop-if-true
    n208 = Get Queue Status(queue=w387) -> (queue out=w383:refnum<queue>, # elements in queue=w382:i32)  [unwired: 2 in, 6 out]
    n209 = Wait (ms)(milliseconds to wait=u32 1000 ("等待时间（毫秒）")) -> ()  [unwired: 1 out]
    n210 = case shown="0" w382 {
      tunnel: w383 -> [_ w390]
      frame Default {
      }
      frame 0 {
        w399 = u16 2 items=["总磷"=1, "总氮"=2, "氨氮"=3] ("站号")
        # "试剂填充 172 \n管路清洗108\n氨氮92\n总磷131\n总磷海水147\n总氮76\n总氮海水92"
        n211 = Bundle By Name(cluster=cluster{"命令":string, "data":variant} {"命令"="", "data"=variant} ("元素"), "命令"="读状态告警区", "data"=w399) -> (w405:cluster{"命令":string, "data":variant})
        n212 = Bundle By Name(cluster=cluster{"命令":string, "data":variant} {"命令"="", "data"=variant} ("元素"), "命令"="读测量数据区", "data"=w399) -> (w402:cluster{"命令":string, "data":variant})
        n213 = global read "VAR总氮全局变量.vi" "状态告警区"() -> (w391:T8)
        n214 = Unbundle By Name(w391) -> ("系统时间"=w398:timestamp)
        n215 = Enqueue Element(queue=w390, element=w405) -> (queue out=w400:refnum<queue>)  [unwired: 2 in, 2 out]
        n216 = Get Date/Time In Seconds() -> (seconds since 1Jan1904=w397:timestamp)
        n217 = Subtract(x=w397, y=w398) -> (x-y=w396:dbl)
        n218 = Absolute Value(x=w396) -> (abs(x)=w395:dbl)
        n219 = Enqueue Element(queue=w400, element=w402) -> (queue out=w392:refnum<queue>)  [unwired: 2 in, 2 out]
        n220 = Greater Or Equal?(x=w395, y=120.0) -> (x >= y?=w393:bool)
        n221 = case shown="真" w393 {
          tunnel: w392 -> [_ w408]
          frame False {
          }
          frame True {
            n222 = call "总氮启动命令.vi"("参数"=T18 {"站号"=3, "量程切换"=enum."AUTO", "控制命令"=enum."校时", "模式设置"=enum."待机", "测量间隔"=0}) -> ("启动命令"=w407:cluster{"命令":string, "data":variant})  [unwired: 10 in]
            n223 = Enqueue Element(queue=w408, element=w407) -> ()  [unwired: 2 in, 3 out]
          }
        }
      }
    }
    n224 = global read "总氮断电保存全局变量.vi" "流程路径"() -> (w386:path)
    n225 = global read "总氮断电保存全局变量.vi" "MB通信方式选择"() -> (w384:enum16{"串口", "TCP"})
    n226 = local write "流程路径"(w386) -> ()
    n227 = case shown="\"TCP\"" w384 {
      tunnel: [w410 w411] -> w385
      frame "串口", Default {
        n228 = global read "总氮断电保存全局变量.vi" "VISA Resource"() -> (w410:refnum<visa-resource-name>)
      }
      frame "TCP" {
        n229 = global read "总氮断电保存全局变量.vi" "IP"() -> (w411:string)
      }
    }
    "字符串" <- w385
  }
  n230 = while {
    tunnel: w24 -> [w418]
    tunnel: w23 -> [w417]
    tunnel: w22 -> [w416]
    tunnel: w21 -> [w415]
    tunnel: w20 -> [w414]
    tunnel: w11 -> [w413]
    tunnel: w15 -> [_]
    tunnel: w12 -> [w412]
    stop <- FALSE stop-if-true
    n231 = event shown="[20] \"写公式\": 值改变" {
      selector: _ -> [_ _ _ _ _ _ _ _ _ _ _ _ _ _ _ _ _ _ _ _ _ _ _]
      dyn-events: _ -> [_ _ _ _ _ _ _ _ _ _ _ _ _ _ _ _ _ _ _ _ _ _ _]
      timeout: _ -> [_ _ _ _ _ _ _ _ _ _ _ _ _ _ _ _ _ _ _ _ _ _ _]
      tunnel: w418 -> [_ _ _ _ w438 w452 _ _ _ _ _ _ w512 _ w522 w557 _ _ _ _ _ _ _]
      tunnel: w417 -> [_ _ _ _ _ _ _ _ _ _ _ _ _ _ _ _ _ _ _ w573 _ _ _]
      tunnel: w416 -> [_ _ _ _ _ _ _ _ _ _ _ _ _ _ _ _ _ _ _ w571 _ w603 w610]
      tunnel: w415 -> [_ _ _ _ _ _ _ _ _ _ _ _ _ _ _ _ _ _ _ w572 _ _ _]
      tunnel: w414 -> [_ _ _ _ _ _ _ _ _ _ _ _ _ _ _ _ _ _ _ w567 _ _ _]
      tunnel: w413 -> [_ _ _ _ _ _ _ _ _ _ _ _ _ _ _ _ _ _ _ _ _ w601 _]
      tunnel: w412 -> [_ _ _ _ _ _ _ _ _ _ _ _ _ _ _ w553 _ _ _ _ _ _ _]
      tunnel: [_ _ _ w424 _ _ _ _ _ _ _ _ _ _ _ _ _ _ _ _ _ _ _] -> _
      event Timeout {
        n232 = event-data() -> ()  [unwired: 1 in, 3 out]
      }
      event "流程固件": Value Change {
        # "试剂填充 172 \n管路清洗108\n氨氮92\n总磷131\n总磷海水147\n总氮76\n总氮海水92"
        n233 = event-data() -> ()  [unwired: 1 in, 6 out]
        n234 = call "流程固件设置对话框.vi"() -> ()  [unwired: 12 in]
      }
      event "布尔": Mouse Down {
        n235 = event-data() -> ("CtlRef"=w421:refnum<vi>)  [unwired: 1 in, 5 out]
        n236 = property class="Bool (严格)"(reference=w421) -> ("Value"=w420:bool)  [unwired: 1 in, 2 out]
        n237 = case shown="假" w420 {
          frame False {
            n238 = call "密码键盘.vi"() -> ("NewNumber"=→"输入密码":dbl)  [unwired: 1 in]
          }
          frame True {
            n239 = local write "输入密码"(u32 0 ("输入密码")) -> ()
          }
        }
      }
      event "测量模式下拉列表", "量程下拉列表", "参数下拉列表": Value Change {
        n240 = event-data() -> ()  [unwired: 1 in, 6 out]
        n241 = local read "测量模式下拉列表"() -> (w426:enum16{"水样测量", "零点核查", "跨度核查", "标样核查", "加标回收"})
        n242 = local read "参数下拉列表"() -> (w425:enum16{"总磷", "总氮"})
        n243 = local read "量程下拉列表"() -> (w427:enum16{"低量程", "高量程"})
        n244 = Bundle("参数下拉列表"=w425, "测量模式下拉列表"=w426, "量程下拉列表"=w427) -> (w428:T12)  [unwired: 1 in]
        n245 = property on="曲线模型" class="曲线模型 (严格)"("属性"=w428) -> (error out=w424:errorcluster)  [unwired: 2 in, 1 out]
      }
      event "串口设置": Value Change {
        n246 = event-data() -> ()  [unwired: 1 in, 6 out]
        n247 = global read "总氮断电保存全局变量.vi" "MB通信方式选择"() -> (w429:enum16{"串口", "TCP"})
        n248 = global read "总氮断电保存全局变量.vi" "VISA Resource"() -> (w435:refnum<visa-resource-name>)
        n249 = global read "总氮断电保存全局变量.vi" "PORT"() -> (w434:string)
        n250 = global read "总氮断电保存全局变量.vi" "IP"() -> (w430:string)
        n251 = call "串口配置.vi"("PORT"=w434, "IP"=w430, "MB通信方式选择"=w429, "请选择串口:"=w435) -> ("PORT 2"=w432:string, "IP 2"=w433:string, "确认 2"=w436:bool, "VISA资源名称 2"=w437:refnum<visa-resource-name>, "MB通信方式选择 2"=w431:enum16{"串口", "TCP"})  [unwired: 3 in]
        n252 = case shown="真" w436 {
          tunnel: w437 -> [_ w443]
          tunnel: w438 -> [_ w442]
          tunnel: w433 -> [_ w441]
          tunnel: w432 -> [_ w440]
          tunnel: w431 -> [_ w439]
          frame False {
          }
          frame True {
            n253 = flat-sequence {
              tunnel: w443 -> [w448]
              tunnel: w442 -> [w449]
              tunnel: w441 -> [w447]
              tunnel: w440 -> [w446]
              tunnel: w439 -> [w445]
              frame #0 {
                n254 = global write "总氮断电保存全局变量.vi" "IP"(w447) -> ()
                n255 = global write "总氮断电保存全局变量.vi" "PORT"(w446) -> ()
                n256 = global write "总氮断电保存全局变量.vi" "VISA Resource"(w448) -> ()
                n257 = global write "总氮断电保存全局变量.vi" "MB通信方式选择"(w445) -> ()
                n258 = Flush Queue(queue=w449) -> (queue out=w444:refnum<queue>)  [unwired: 1 in, 2 out]
                n259 = Enqueue Element(queue=w444, element=cluster{"命令":string, "data":variant} {"命令"="启用模块", "data"=variant} ("元素")) -> ()  [unwired: 2 in, 3 out]
              }
              frame #1 {
                n260 = call "配置文件保存.vi"() -> ()  [unwired: 12 in]
              }
            }
          }
        }
      }
      event "模块启用": Value Change {
        n261 = event-data() -> ("OldVal"=w453:bool)  [unwired: 1 in, 5 out]
        n262 = Flush Queue(queue=w452) -> (queue out=w451:refnum<queue>)  [unwired: 1 in, 2 out]
        n263 = case shown="假" w453 {
          tunnel: w451 -> [w454 w456]
          frame False {
            n264 = Enqueue Element(queue=w454, element=cluster{"命令":string, "data":variant} {"命令"="停用模块", "data"=variant} ("元素")) -> ()  [unwired: 2 in, 3 out]
          }
          frame True {
            n265 = Enqueue Element(queue=w456, element=cluster{"命令":string, "data":variant} {"命令"="启用模块", "data"=variant} ("元素")) -> ()  [unwired: 2 in, 3 out]
          }
        }
      }
      event "流程路径": Value Change {
        n266 = event-data() -> ()  [unwired: 1 in, 6 out]
        n267 = flat-sequence {
          frame #0 {
            n268 = local read "流程路径"() -> (w458:path)
            n269 = global write "总氮断电保存全局变量.vi" "流程路径"(w458) -> ()
          }
          frame #1 {
            n270 = call "配置文件保存.vi"() -> ()  [unwired: 12 in]
          }
        }
      }
      event "公式一键写入": Value Change {
        n271 = event-data() -> ()  [unwired: 1 in, 6 out]
        n272 = local read "公式"() -> (w459:cluster{"X^2":dbl, "X":dbl, "b":dbl})
        n273 = call "公式复合写入.vi"("公式"=w459) -> ()  [unwired: 11 in]
      }
      event "曲线模型": Value Change {
        n274 = event-data() -> ()  [unwired: 1 in, 6 out]
        n275 = Unbundle By Name("曲线模型") -> ("X^2"=w462:dbl, "X"=w463:dbl, "B"=w464:dbl)
        n276 = Build Array(w462, w463, w464) -> (w461:dbl[])
        n277 = Array To Cluster(array=w461) -> (cluster=w460:cluster{"[0]":dbl, "[1]":dbl, "[2]":dbl})
        n278 = local write "公式"(w460) -> ()
      }
      event "质控参数设置": Value Change {
        n279 = event-data() -> ()  [unwired: 1 in, 6 out]
        n280 = global read "总氮断电保存全局变量.vi" "质控参数设置"() -> (w466:T19)
        n281 = call "总氮质控参数设置.vi"("质控参数设置"=w466) -> ("输出簇"=w467:T20)  [unwired: 10 in]
        n282 = Unbundle By Name(w467) -> ("确定"=w468:bool)
        n283 = case shown="真" w468 {
          tunnel: w467 -> [_ w470]
          tunnel: w466 -> [_ w469]
          frame False {
          }
          frame True {
            n284 = flat-sequence {
              tunnel: w470 -> [w477]
              tunnel: w469 -> [w476]
              frame #0 {
                n285 = Unbundle By Name(w477) -> ("跨度值"=w475:dbl, "零点标准液浓度"=w474:dbl, "跨度标准液浓度"=w473:dbl, "标准液标准浓度"=w472:dbl)
                n286 = Bundle By Name(cluster=w476, "跨度值"=w475, "零点标准液浓度"=w474, "跨度标准液浓度"=w473, "标准液标准浓度"=w472) -> (w471:T19)
                n287 = global write "总氮断电保存全局变量.vi" "质控参数设置"(w471) -> ()
              }
              frame #1 {
                n288 = call "配置文件保存.vi"() -> ()  [unwired: 12 in]
              }
            }
          }
        }
      }
      event "仪器参数设置": Value Change {
        n289 = event-data() -> ()  [unwired: 1 in, 6 out]
        n290 = global read "总氮断电保存全局变量.vi" "总氮仪器参数"() -> (w478:T21)
        n291 = call "仪器参数设置.vi"("氨氮仪器参数"=w478) -> ("仪器参数设置输出"=w479:T22)  [unwired: 10 in]
        n292 = Unbundle By Name(w479) -> ("确定"=w480:bool)
        n293 = case shown="真" w480 {
          tunnel: w479 -> [_ w482]
          tunnel: w478 -> [_ w481]
          frame False {
          }
          frame True {
            n294 = flat-sequence {
              tunnel: w482 -> [w499]
              tunnel: w481 -> [w498]
              frame #0 {
                n295 = Unbundle By Name(w499) -> ("测量量程"=w497:dbl, "测量精度"=w496:dbl, "测量间隔"=w495:dbl, "消解温度"=w494:dbl, "消解时长"=w492:dbl, "空白校准时间"=w491:timestamp, "曲线截距"=w490:dbl, "曲线斜率"=w489:dbl, "测量检出限"=w488:dbl, "测量信号值"=w487:dbl, "线性相关系数"=w486:dbl, "二次多项式系数"=w485:dbl, "标样校准时间"=w484:timestamp, "稀释倍数"=w483:dbl)
                n296 = Bundle By Name(cluster=w498, "测量量程"=w497, "测量精度"=w496, "测量间隔"=w495, "消解温度"=w494, "消解时长"=w492, "空白校准时间"=w491, "曲线截距"=w490, "曲线斜率"=w489, "测量检出限"=w488, "测量信号值"=w487, "线性相关系数"=w486, "二次多项式系数"=w485, "标样校准时间"=w484, "稀释倍数"=w483) -> (w493:T21)
                n297 = global write "总氮断电保存全局变量.vi" "总氮仪器参数"(w493) -> ()
              }
              frame #1 {
                n298 = call "配置文件保存.vi"() -> ()  [unwired: 12 in]
              }
            }
          }
        }
      }
      event "自动测试量程配置": Value Change {
        n299 = event-data() -> ()  [unwired: 1 in, 6 out]
        n300 = flat-sequence {
          frame #0 {
            n301 = global write "总氮断电保存全局变量.vi" "总氮自动测试量程配置"("自动测试量程配置") -> ()
          }
          frame #1 {
            n302 = call "配置文件保存.vi"() -> ()  [unwired: 12 in]
          }
        }
      }
      event "手动启动": Value Change {
        n303 = event-data() -> ()  [unwired: 1 in, 6 out]
        n304 = call "总氮启动参数对话框.vi"() -> ("标样浓度输出"=w501:dbl, "确认"=w511:bool, "元素"=w503:cluster{"命令":string, "data":variant})  [unwired: 9 in]
        n305 = case shown="真" w511 {
          tunnel: w512 -> [_ w518]
          tunnel: w503 -> [_ w517]
          frame False {
          }
          frame True {
            n306 = Enqueue Element(queue=w518, element=w517) -> ()  [unwired: 2 in, 3 out]
          }
        }
        n307 = Unbundle By Name(w503) -> ("data"=w509:variant)
        n308 = Variant To Data(type=cluster{"站号":u16, "控制命令":u16[]} {"站号"=0, "控制命令"=[]} ("输出簇"), Variant=w509) -> (data=w508:cluster{"站号":u16, "控制命令":u16[]})  [unwired: 1 in, 1 out]
        n309 = Unbundle By Name(w508) -> ("控制命令"=w507:u16[])
        n310 = Index Array(array=w507) -> (element=w506:u16)  [unwired: 1 in]
        n311 = Swap Bytes(anything=w506) -> (byte swapped=w505:u16)
        n312 = Equal?(x=w505, y=u16 2) -> (x = y?=w502:bool)
        n313 = case shown="真" w502 {
          tunnel: w501 -> [_ w513]
          frame False {
          }
          frame True {
            n314 = flat-sequence {
              tunnel: w513 -> [w515]
              frame #0 {
                n315 = global read "总氮断电保存全局变量.vi" "质控参数设置"() -> (w516:T19)
                n316 = Bundle By Name(cluster=w516, "标准液标准浓度"=w515) -> (w514:T19)
                n317 = global write "总氮断电保存全局变量.vi" "质控参数设置"(w514) -> ()
              }
              frame #1 {
                n318 = call "配置文件保存.vi"() -> ()  [unwired: 12 in]
              }
            }
          }
        }
      }
      event "单步测试": Value Change {
        n319 = event-data() -> ()  [unwired: 1 in, 6 out]
        n320 = call "总氮单步调试对话框.vi"() -> ()  [unwired: 12 in]
      }
      event "校准按钮.校准1", "校准按钮.校准2", "校准按钮.校准3", "校准按钮.校准4", "校准按钮.校准5": Value Change {
        n321 = event-data() -> ("CtlRef"=w528:refnum<vi>)  [unwired: 1 in, 5 out]
        n322 = property class="Bool"(reference=w528) -> ("Label.Text"=w526:string)  [unwired: 1 in, 2 out]
        n323 = property on="曲线模型" class="曲线模型 (严格)"() -> ("浓度属性"=w527:T23)  [unwired: 2 in, 2 out]
        n324 = case shown="\"校准3\"" w526 {
          tunnel: [w536 w539 w542 w545 w548] -> w524
          tunnel: [u16 1 ("校准点1-5") u16 2 ("校准点1-5") u16 3 ("校准点1-5") u16 4 ("校准点1-5") u16 5 ("校准点1-5")] -> w525
          tunnel: w527 -> [w537 w540 w543 w546 w549]
          frame "校准1", Default {
            n325 = Unbundle By Name(w537) -> ("标液浓度1"=w536:dbl)
          }
          frame "校准2" {
            n326 = Unbundle By Name(w540) -> ("标液浓度2"=w539:dbl)
          }
          frame "校准3" {
            n327 = Unbundle By Name(w543) -> ("标液浓度3"=w542:dbl)
          }
          frame "校准4" {
            n328 = Unbundle By Name(w546) -> ("标液浓度4"=w545:dbl)
          }
          frame "校准5" {
            n329 = Unbundle By Name(w549) -> ("标液浓度5"=w548:dbl)
          }
        }
        n330 = local read "量程下拉列表"() -> (w519:enum16{"低量程", "高量程"})
        n331 = Not Equal To 0?(x=w524) -> (x != 0?=w520:bool)
        n332 = Bundle By Name(cluster=cluster{"校准？":bool, "校准点1-5":u16, "校准浓度":dbl} {"校准？"=FALSE, "校准点1-5"=0, "校准浓度"=0.0} ("校准输出"), "校准？"=TRUE, "校准点1-5"=w525, "校准浓度"=w524) -> (w523:cluster{"校准？":bool, "校准点1-5":u16, "校准浓度":dbl})
        n333 = case shown="真" w520 {
          tunnel: [cluster{"命令":string, "data":variant} {"命令"="启动", "data"=variant(cluster{"站号":u16, "控制命令":u16[]} {"站号"=2, "控制命令"=[2048, 256]})} ("元素") w532] -> w521
          tunnel: w519 -> [_ w533]
          frame False {
            # "校零"
          }
          frame True {
            # "校标"
            n334 = case shown="\"低量程\", 默认" w533 {
              tunnel: [cluster{"命令":string, "data":variant} {"命令"="启动", "data"=variant(cluster{"站号":u16, "控制命令":u16[]} {"站号"=2, "控制命令"=[2304, 256]})} ("元素") cluster{"命令":string, "data":variant} {"命令"="启动", "data"=variant(cluster{"站号":u16, "控制命令":u16[]} {"站号"=2, "控制命令"=[2304, 257]})} ("元素")] -> w532
              frame "低量程", Default {
              }
              frame "高量程" {
              }
            }
          }
        }
        n335 = global write "总氮断电保存全局变量.vi" "校准输出"(w523) -> ()
        n336 = Enqueue Element(queue=w522, element=w521) -> ()  [unwired: 2 in, 3 out]
      }
      event "停止": Value Change {
        n337 = event-data() -> ()  [unwired: 1 in, 6 out]
        n338 = Enqueue Element(queue=w557, element=cluster{"命令":string, "data":variant} {"命令"="启动", "data"=variant(cluster{"站号":u16, "控制命令输出":u16[]} {"站号"=1, "控制命令输出"=[2816]})} ("元素")) -> (queue out=w554:refnum<queue>)  [unwired: 2 in, 2 out]
        n339 = Cancel Notification(0:w553) -> (8:w552:refnum<notifier>)  [unwired: 1 in, 2 out]
        n340 = Send Notification(notification=TRUE ("通知"), notifier=w552) -> ()  [unwired: 1 in, 2 out]
        n341 = Enqueue Element(queue=w554, element=cluster{"命令":string, "data":variant} {"命令"="启动", "data"=variant(cluster{"站号":u16, "控制命令输出":u16[]} {"站号"=2, "控制命令输出"=[2816]})} ("元素")) -> ()  [unwired: 2 in, 3 out]
      }
      event "设置": Value Change {
        n342 = event-data() -> ()  [unwired: 1 in, 6 out]
        n343 = property on="窗格" class="Pane"("Origin"=T7 {"Horizontal"=0, "Vertical"=628} ("原点")) -> ()  [unwired: 2 in, 2 out]
      }
      event "返回": Value Change {
        n344 = event-data() -> ()  [unwired: 1 in, 6 out]
        n345 = property on="窗格" class="Pane"("Origin"=T7 {"Horizontal"=0, "Vertical"=0} ("原点")) -> ()  [unwired: 2 in, 2 out]
      }
      event "公式.X^2", "公式.X", "公式.b": Mouse Down {
        n346 = event-data() -> ("CtlRef"=w563:refnum<vi>)  [unwired: 1 in, 5 out]
        n347 = property class="DigNum (严格)"(reference=w563) -> (reference out=w561:refnum<vi>, "Value"=w562:dbl)  [unwired: 1 in, 1 out]
        n348 = call "数字键盘.vi"("OldNumber"=w562) -> ("NewNumber"=w560:dbl)
        n349 = property class="DigNum (严格)"(reference=w561, "Val(Sgnl)"=w560) -> ()  [unwired: 1 in, 2 out]
      }
      event "读公式": Value Change {
        n350 = event-data() -> ()  [unwired: 1 in, 6 out]
        n351 = property class="Enum (严格)"(reference=w571) -> ("Value"=w570:enum16{"总磷", "总氮"})  [unwired: 1 in, 2 out]
        n352 = property class="Enum (严格)"(reference=w572) -> ("Value"=w569:enum16{"水样测量", "零点核查", "跨度核查", "标样核查", "加标回收"})  [unwired: 1 in, 2 out]
        n353 = property class="Enum (严格)"(reference=w573) -> ("Value"=w568:enum16{"低量程", "高量程"})  [unwired: 1 in, 2 out]
        n354 = call "总磷总氮公式读取.vi"("量程"=w568, "测量模式"=w569, "测量参数"=w570) -> ("error out"=w565:errorcluster, "公式"=w566:cluster{"X^2":dbl, "X":dbl, "b":dbl})  [unwired: 7 in]
        n355 = property class="Clust (严格)"(reference=w567, "Value"=w566) -> ()  [unwired: 1 in, 2 out]
        n356 = case shown="错误" w565 {
          tunnel: ["读取成功" ("消息") "读取失败" ("消息")] -> w564
          frame No Error {
          }
          frame Error {
          }
        }
        n357 = One Button Dialog(message=w564) -> ()  [unwired: 1 in, 1 out]
      }
      event "写公式": Value Change {
        n358 = event-data() -> ()  [unwired: 1 in, 6 out]
        n359 = call "总磷总氮公式写入.vi"("公式"="公式", "量程"="量程下拉列表", "测量模式"="测量模式下拉列表", "测量参数"="参数下拉列表") -> ("error out"=w580:errorcluster)  [unwired: 7 in]
        n360 = case shown="无错误" w580 {
          tunnel: ["写入成功" ("消息") "写入失败" ("消息")] -> w581
          tunnel: "测量模式下拉列表" -> [w584 _]
          tunnel: "量程下拉列表" -> [w583 _]
          tunnel: "公式" -> [w582 _]
          frame No Error {
            n361 = Equal?(x=w584, y=enum16{"水样测量", "零点核查", "跨度核查", "标样核查", "加标回收"}."水样测量") -> (x = y?=w587:bool)
            n362 = Equal?(x=w583, y=enum16{"低量程", "高量程"}."低量程") -> (x = y?=w586:bool)
            n363 = Compound Arithmetic op=AND ("复合运算")(w587, w586) -> (w585:bool)
            n364 = case shown="真" w585 {
              tunnel: w582 -> [_ w596]
              frame False {
              }
              frame True {
                n365 = Unbundle By Name(w596) -> ("X^2"=w593:dbl, "X"=w595:dbl, "b"=w594:dbl)
                n366 = global read "总氮断电保存全局变量.vi" "总氮仪器参数"() -> (w592:T21)
                n367 = Bundle By Name(cluster=w592, "曲线截距"=w594, "曲线斜率"=w595, "二次多项式系数"=w593) -> (w591:T21)
                n368 = global write "总氮断电保存全局变量.vi" "总氮仪器参数"(w591) -> ()
              }
            }
          }
          frame Error {
          }
        }
        n369 = One Button Dialog(message=w581) -> ()  [unwired: 1 in, 1 out]
      }
      event "量程切换阈值读取": Value Change {
        n370 = event-data() -> ()  [unwired: 1 in, 6 out]
        n371 = property class="Enum (严格)"(reference=w603) -> ("Value"=w602:enum16{"总磷", "总氮"})  [unwired: 1 in, 2 out]
        n372 = call "总磷总氮量程读取.vi"("测量参数"=w602) -> ("error out"=w598:errorcluster, "量程参数读取"=w600:T24)  [unwired: 9 in]
        n373 = property class="Clust (严格)"(reference=w601, "Value"=w600) -> ()  [unwired: 1 in, 2 out]
        n374 = case shown="错误" w598 {
          tunnel: ["读取成功" ("消息") "读取失败" ("消息")] -> w599
          frame No Error {
          }
          frame Error {
          }
        }
        n375 = One Button Dialog(message=w599) -> ()  [unwired: 1 in, 1 out]
      }
      event "量程切换阈值写入": Value Change {
        n376 = event-data() -> ()  [unwired: 1 in, 6 out]
        n377 = property class="Enum (严格)"(reference=w610) -> ("Value"=w609:enum16{"总磷", "总氮"})  [unwired: 1 in, 2 out]
        n378 = call "总磷总氮量程写入.vi"("量程参数写入"="量程参数读取", "测量参数"=w609) -> ("error out"=w607:errorcluster)  [unwired: 8 in]
        n379 = case shown="无错误" w607 {
          tunnel: ["写入成功" ("消息") "写入失败" ("消息")] -> w608
          frame No Error {
          }
          frame Error {
          }
        }
        n380 = One Button Dialog(message=w608) -> ()  [unwired: 1 in, 1 out]
      }
    }
  }
  n381 = while {
    tunnel: [w620] -> _
    shift-right: [w618] -> _
    shift-left: w5 -> [w617]
    tunnel: w1 -> [w614]
    stop <- FALSE stop-if-true
    n382 = global read "VAR总氮全局变量.vi" "配置文件 path"() -> (w613:path)
    n383 = Wait (ms)(milliseconds to wait=u32 1000 ("等待时间（毫秒）")) -> ()  [unwired: 1 out]
    n384 = Read from Text File(file (use dialog)=w613, error in=w614) -> (text=w618:string, error out=w615:errorcluster)  [unwired: 2 in, 2 out]
    n385 = Not Equal?(x=w618, y=w617) -> (x != y?=w616:bool)
    n386 = case shown="真" w616 {
      tunnel: [w622 w626] -> w620
      tunnel: w613 -> [_ w625]
      tunnel: w615 -> [w622 w624]
      frame False {
      }
      frame True {
        # "文件发生改变进行更新"
        n387 = call <vilib>:"Open Config Data.vi"("error in (no error)"=w624, "configuration file path"=w625) -> ("error out"=w630:errorcluster, "refnum"=w629:T14)  [unwired: 7 in, 1 out]
        n388 = vi-ref "总氮断电保存全局变量.vi"() -> (w623:refnum<vi>)
        n389 = call <userlib>:"Read Panel from INI__ogtk.vi"("error in (no error)"=w630, "VI ref"=w623, "refnum"=w629) -> ("error out"=w628:errorcluster, "refnum out"=w627:T14)  [unwired: 7 in]
        n390 = call <vilib>:"Close Config Data.vi"("error in (no error)"=w628, "refnum"=w627) -> ("error out"=w626:errorcluster)  [unwired: 8 in, 1 out]
      }
    }
  }
  n391 = while {
    stop <- FALSE stop-if-true
    n392 = vi-ref "总氮测量流程.vi"() -> (w640:refnum<vi>)
    n393 = global read "VAR总氮全局变量.vi" "状态告警区"() -> (w634:T8)
    n394 = Wait (ms)(milliseconds to wait=u32 1000 ("等待时间（毫秒）")) -> ()  [unwired: 1 out]
    n395 = Unbundle By Name("定时设置") -> ("启动"=w635:bool, "控制命令"=w636:T1)
    n396 = property class="VI"(reference=w640) -> ("Exec.State"=w638:T25, "Name"=w639:string)  [unwired: 1 in, 2 out]
    n397 = global read "总氮断电保存全局变量.vi" "总氮自动测试量程配置"() -> (w641:T6)
    n398 = case shown="真" w635 {
      tunnel: w639 -> [_ w650]
      tunnel: w636 -> [_ w649]
      tunnel: w638 -> [_ w648]
      frame False {
      }
      frame True {
        n399 = case shown="\"Idle\"" w648 {
          tunnel: w650 -> [_ w654]
          tunnel: w649 -> [_ w652]
          frame "Bad", Default {
          }
          frame "Idle" {
            n400 = Open VI Reference(type specifier VI Refnum (for type only)=refnum<vi> refnum, vi path=w654, options=128 ("选项")) -> (vi reference=w655:refnum<vi>, error out=w656:errorcluster)  [unwired: 3 in]
            n401 = call-by-ref "开始异步调用"(reference=w655, error in=w656, "控制命令"=w652) -> (reference out=w657:refnum<vi>, error out=w658:errorcluster)  [unwired: 11 in]
            n402 = Close Reference(reference=w657, error in (no error)=w658) -> ()  [unwired: 1 out]
          }
        }
      }
    }
    n403 = Unbundle By Name(w634) -> ("工作状态"=w633:T10)
    n404 = case shown="\"空闲\"" w633 {
      tunnel: [_ TRUE] -> w631
      frame "空闲" {
      }
      frame "水样测试", Default {
      }
    }
    n405 = local write "自动测试量程配置"(w641) -> ()
    n406 = property on="定时设置" class="定时设置 (严格)"("仪器状态"=w631) -> ("是否重写配置文件"=w632:bool)  [unwired: 2 in, 2 out]
    n407 = case shown="真" w632 {
      frame False {
        n408 = global read "总氮断电保存全局变量.vi" "定时配置信息"() -> (w644:cluster{"周期模式":T26, "定点周期":T27, "间隔启动":T29})
        n409 = property on="定时设置" class="定时设置 (严格)"("配置信息"=w644) -> ()  [unwired: 2 in, 2 out]
      }
      frame True {
        n410 = flat-sequence {
          frame #0 {
            n411 = property on="定时设置" class="定时设置 (严格)"() -> ("配置信息"=w645:cluster{"周期模式":T26, "定点周期":T27, "间隔启动":T29})  [unwired: 2 in, 2 out]
            n412 = global write "总氮断电保存全局变量.vi" "定时配置信息"(w645) -> ()
          }
          frame #1 {
            n413 = call "配置文件保存.vi"() -> ()  [unwired: 12 in]
          }
          frame #2 {
            n414 = property on="定时设置" class="定时设置 (严格)"("是否重写配置文件"=FALSE) -> ()  [unwired: 2 in, 2 out]
          }
        }
      }
    }
  }
  n415 = call "Create balloon 队列.vi"() -> ("队列输出"=w2:refnum<queue>)  [unwired: 11 in]
  n416 = while {
    tunnel: w2 -> [w659]
    stop <- FALSE stop-if-true
    n417 = global read "VAR总氮全局变量.vi" "状态告警区"() -> (w665:T8)
    n418 = Unbundle By Name(w665) -> ("id"=w664:u16, "告警代码"=w663:u16, "故障代码"=w662:u16)
    n419 = while {
      tunnel: w664 -> [w678]
      tunnel: w663 -> [w668]
      tunnel: w662 -> [w667]
      shift-right: [w667] -> _
      shift-left: _ -> [w673]
      shift-right: [w668] -> _
      shift-left: _ -> [w672]
      tunnel: w659 -> [w666]
      stop <- TRUE stop-if-true
      n420 = Not Equal?(x=w672, y=w668) -> (x != y?=w670:bool)
      n421 = Not Equal?(x=w673, y=w667) -> (x != y?=w671:bool)
      n422 = Not Equal To 0?(x=w668) -> (x != 0?=w676:bool)
      n423 = Not Equal To 0?(x=w667) -> (x != 0?=w675:bool)
      n424 = Or(x=w676, y=w675) -> (x .or. y?=w674:bool)
      n425 = Or(x=w670, y=w671) -> (x .or. y?=w669:bool)
      n426 = case shown="真" w669 {
        tunnel: w678 -> [_ w683]
        tunnel: w674 -> [_ w682]
        tunnel: w668 -> [_ w681]
        tunnel: w667 -> [_ w680]
        tunnel: w666 -> [_ w679]
        frame False {
        }
        frame True {
          n427 = case shown="真" w682 {
            tunnel: w683 -> [_ w698]
            tunnel: w681 -> [_ w697]
            tunnel: w680 -> [_ w696]
            tunnel: w679 -> [_ w688]
            frame False {
            }
            frame True {
              n428 = call "故障码字段定义.vi"("故障代码"=w696) -> ("字符串"=w686:string)  [unwired: 10 in]
              n429 = call "告警码字段定义.vi"("告警代码"=w697) -> ("故障详情"=w684:string, "通用告警信息"=w690:string, "字符串"=w685:string)  [unwired: 8 in]
              n430 = Format Into String(format string="【%s】%s" ("格式字符串"), initial string="" ("初始字符串"), w686, w690) -> (resulting string=w693:string)  [unwired: 1 in, 1 out]
              n431 = call "id参数转换.vi"("id"=w698) -> ("table输出"=w687:string)  [unwired: 10 in]
              n432 = Search and Replace String(replace all?=TRUE ("替换全部？(F)"), input string=w693, search string="【无故障】|无告警" ("字符串")) -> (result string=w689:string)  [unwired: 5 in, 3 out]
              n433 = Get Date/Time In Seconds() -> (seconds since 1Jan1904=w701:timestamp)
              n434 = call "balloon入队列.vi"("队列"=w688, "故障详情"=w684, "告警信息"=w685, "故障信息"=w686, "参数名称"=w687) -> ()  [unwired: 6 in, 1 out]
              n435 = Bundle By Name(cluster=T30 {"时间标识"=timestamp(0 s since 1904-01-01), "设备"="", "日志信息"="", "备注"=""} ("data in"), "时间标识"=w701, "设备"=w687, "日志信息"=w689, "备注"=w684) -> (w699:T30)
              n436 = call "总氮报警信息.vi"("data in"=w699) -> ()  [unwired: 10 in, 1 out]
            }
          }
        }
      }
    }
    n437 = Wait (ms)(milliseconds to wait=u32 100 ("等待时间（毫秒）")) -> ()  [unwired: 1 out]
  }
